vi "Get Image Number of Pixel Values.vi"(8 "Error In":errorcluster, 11 "Image":T1) -> (0 "Error Out":errorcluster, 1 "# Distinct Pixel Values":i32, 3 "Pixel Values":i32[](array[numeric]))   [LabVIEW 2021, in "Image.lvlib"]
uses:
  <vilib>/vision/Image Controls.llb/IMAQ Image.ctl
  Image.lvlib
  <vilib>/vision/NI_Vision_Development_Module.lvlib
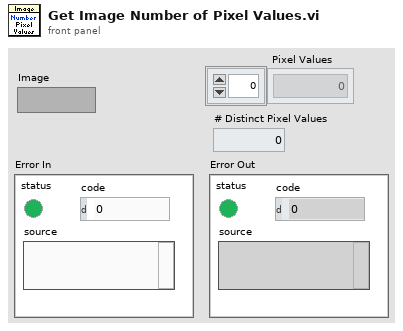
[diagram p1: front panel]
types:
  T1 = typedef "IMAQ Image.ctl" = refnum<image>
  T2 = typedef "Image Type" = u32
  T3 = cluster{"histogram":u32[], "Minimal Value":sgl, "Maximal Value":sgl, "Starting Value":sgl, "Interval Width":sgl, "Mean Value":sgl, "Standard  Variation":sgl, "Area (pixels)":i32}
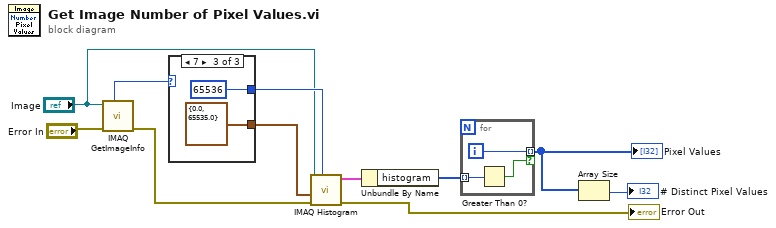
[diagram p0: block diagram]
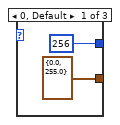
[diagram p2: hidden frame]
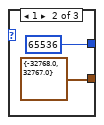
[diagram p3: hidden frame]
diagram:
  n1 = call "IMAQ GetImageInfo"("error in (no error)"="Error In", "Image"="Image") -> ("error out"=w5:errorcluster, "Image Type"=w10:T2)  [unwired: 8 out]
  n2 = case shown="7" w10 {
    tunnel: [256 ("Number of Classes") 65536 ("Number of Classes") 65536 ("Number of Classes")] -> w9
    tunnel: [cluster{"Minimum":sgl, "Maximum":sgl} {"Minimum"=0.0, "Maximum"=255.0} ("Interval Range") cluster{"Minimum":sgl, "Maximum":sgl} {"Minimum"=-32768.0, "Maximum"=32767.0} ("Interval Range") cluster{"Minimum":sgl, "Maximum":sgl} {"Minimum"=0.0, "Maximum"=65535.0} ("Interval Range")] -> w8
    frame 0, Default {
    }
    frame 1 {
    }
    frame 7 {
    }
  }
  n3 = call "IMAQ Histogram"("Number of Classes"=w9, "error in (no error)"=w5, "Interval Range"=w8, "Image"="Image") -> ("error out"=→"Error Out":errorcluster, "Histogram Report"=w11:T3)  [unwired: 1 in, 5 out]
  n4 = Unbundle By Name(w11) -> ("histogram"=w3:u32[])
  n5 = for {
    tunnel: w3 -> [w20] mode=indexing
    tunnel: [w19] -> w1 mode=indexing if=w18
    i -> [w19]
    n6 = Greater Than 0?(x=w20) -> (x > 0?=w18:bool)
  }
  "Pixel Values" <- w1
  n7 = Array Size(array=w1) -> (size(s)=→"# Distinct Pixel Values":i32)
